vi "Play Audio.vi"(7 "Audio CFG in":T1 {"task ID" format="%.0x"}, 8 "error in (no error)":errorcluster) -> (0 "error out":errorcluster, 2 "Now Playing":waveform(i16)[](array[waveform]), 3 "Completed ?":bool, 4 "Now Playing (%)":dbl, 5 "Audio CFG out":T1 {"task ID" format="%.0x"}, 6 "Now Playing (Time)":string)   [LabVIEW 2020]
uses:
  typedefs/Audio CFG.ctl
  <vilib>/Dataflow_G/G-Audio/Controls/Audio File Info.ctl
  <vilib>/sound2/lvsound2.llb/Sound Output Task ID.ctl
  d8e7d527-d191-428c-a681-42ea39227684.vi
  <vilib>/Dataflow_G/G-Audio/Private/Get Basic Audio File Info.vi
  <vilib>/Dataflow_G/G-Audio/Private/Result To Error.vi
  d8e7d527-d191-428c-a681-42ea39227684.vi/779dfdfd-1b42-4cf4-8001-66d3dd167625.vi
  d8e7d527-d191-428c-a681-42ea39227684.vi/55d550d4-9624-414e-aebd-6e02b5081896.vi
  Result To Error - Copy.vi
  d8e7d527-d191-428c-a681-42ea39227684.vi/779dfdfd-1b42-4cf4-8001-66d3dd167625.vi/a9d2058a-38f9-4c88-a1a9-9bf864ebbde5.vi
  d8e7d527-d191-428c-a681-42ea39227684.vi/55d550d4-9624-414e-aebd-6e02b5081896.vi/4b7b629c-2e91-4160-9820-a26af8f6e677.vi
  d8e7d527-d191-428c-a681-42ea39227684.vi/55d550d4-9624-414e-aebd-6e02b5081896.vi/e7c4a249-ce38-42b4-8985-5fdb76b4ebfc.vi
  <vilib>/Utility/Data Type/Get Numeric Information.vi
  <vilib>/Utility/error.llb/Error Cluster From Error Code.vi
  <vilib>/sound2/lvsound2.llb/Sound Output Write (I16).vi
  <vilib>/Dataflow_G/G-Audio/G-Audio.lvlib
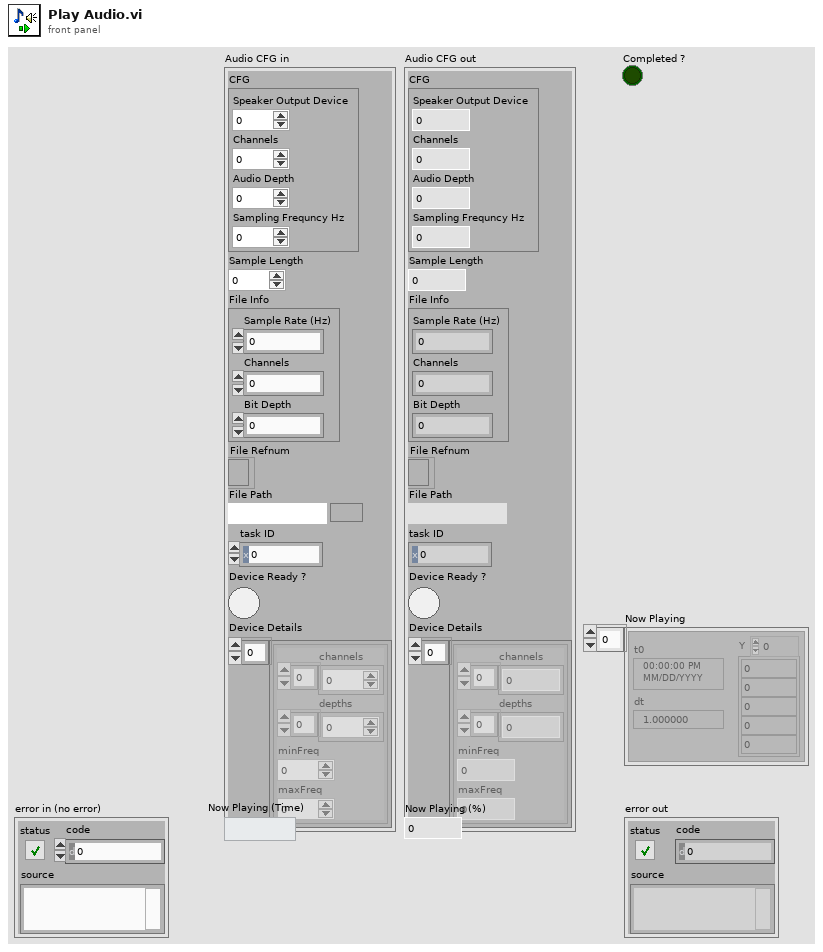
[diagram p1: front panel]
types:
  T1 = typedef "Audio CFG.ctl" = cluster{"CFG":cluster{"Speaker Output Device":u32, "Channels":i32, "Audio Depth":i32, "Sampling Frequncy Hz":dbl}, "Sample Length":u64, "File Info":T2, "File Refnum":refnum<file>, "File Path":path, "Task ID":T3, "Device Ready ?":bool, "Device Details":cluster{"channels":i32[], "depths":i32[], "minFreq":dbl, "maxFreq":dbl}[]}
  T2 = typedef "G-Audio.lvlib/Audio File Info.ctl" = cluster{"Sample Rate (Hz)":u32, "Channels":u32, "Bit Depth":u32}
  T3 = typedef "Sound Output Task ID.ctl" = u32
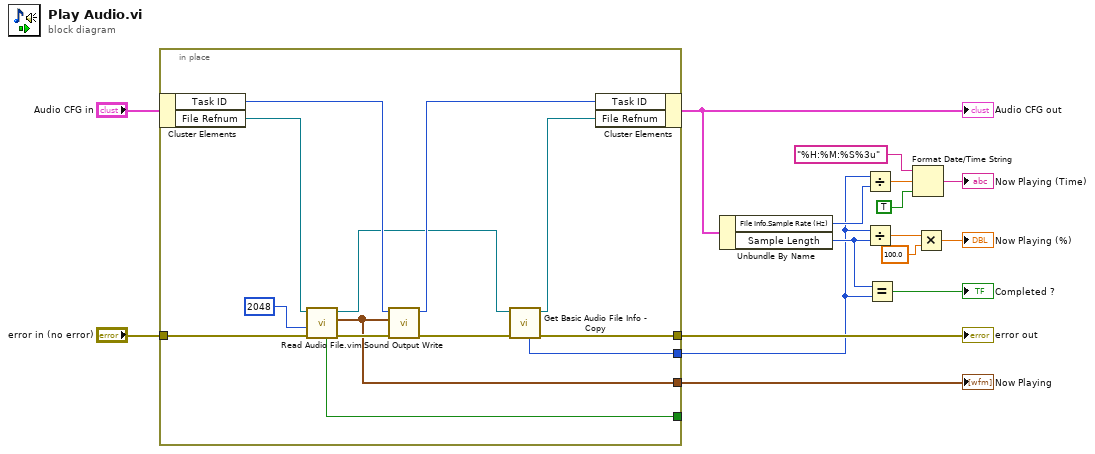
[diagram p0: block diagram]
diagram:
  n1 = in-place {
    in-place-border: "error in (no error)" -> [w29]
    in-place-border: [w22] -> w15
    in-place-border: [w19] -> w2
    in-place-border: [w18] -> _
    in-place-border: [w17] -> w6
    n2 = in-place-cluster #1("Audio CFG in") -> ("Task ID"=w26:T3, "File Refnum"=w27:refnum<file>)
    n3 = call "Read Audio File.vim"("error in (no error)"=w29, "Frames To Read"=u64 2048, "Audio File Refnum In"=w27) -> ("error out"=w28:errorcluster, "Audio Data"=w17:waveform(i16)[], "Audio File Refnum Out"=w23:refnum<file>, "End of File?"=w18:bool)  [unwired: 4 in, 1 out]
    n4 = call-poly <vilib>:"Sound Output Write.vi"("error in (no error)"=w28, "data"=w17, "task ID"=w26) -> ("error out"=w21:errorcluster, "task ID out"=w25:T3)  [unwired: 7 in]
    n5 = call "Get Basic Audio File Info - Copy.vi"("error in (no error)"=w21, "Audio File Refnum In"=w23) -> ("error out"=w22:errorcluster, "Audio File Refnum Out"=w20:refnum<file>, "read_offset"=w19:u64)  [unwired: 5 in, 2 out]
    n6 = in-place-cluster #1("Task ID"=w25, "File Refnum"=w20) -> (w13:T1)
  }
  "Audio CFG out" <- w13
  "error out" <- w15
  "Now Playing" <- w6
  n7 = Unbundle By Name(w13) -> ("File Info.Sample Rate (Hz)"=w8:u32, "Sample Length"=w3:u64)
  n8 = Divide(x=w2, y=w8) -> (x/y=w11:dbl)
  n9 = Divide(x=w2, y=w3) -> (x/y=w7:dbl)
  n10 = Equal?(x=w3, y=w2) -> (x = y?=→"Completed ?":bool)
  n11 = Format Date/Time String(time format string (%c)="%H:%M:%S%3u", seconds (now)=w11, UTC format=TRUE) -> (date/time string=→"Now Playing (Time)":string)
  n12 = Multiply(x=w7, y=100.0) -> (x*y=→"Now Playing (%)":dbl)
